vi "array of clusters.vi"() -> ()   [LabVIEW 2021]
panel:
  in  "array":cluster{"a":dbl}[](array[cluster])=[{"a"=1.0}]
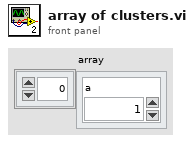
[diagram p1: front panel]
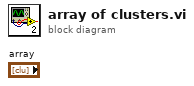
[diagram p0: block diagram]
diagram:
